vi "NodoPropiedad.vi"() -> ()   [LabVIEW 2015]
uses:
  <vilib>/Utility/miscctls.llb/LVPositionTypeDef.ctl
panel:
  out "Position":T1
  in  "Enum":enum16{"Val1", "Val2", "Val3", "Val4"}(ring)
  in  "Cambiar estado lol":T2(ring)
  out "Estado lol":T2(ring)
  in  "stop":bool
  in  "Ver":bool
  in  "Lol":dbl
  out "xd":bool
  in  "Cual desvisivilizar":bool
  in  "This is a Radio Button":enum32{"Option 1", "Option 2", "Option 3"}(radio)
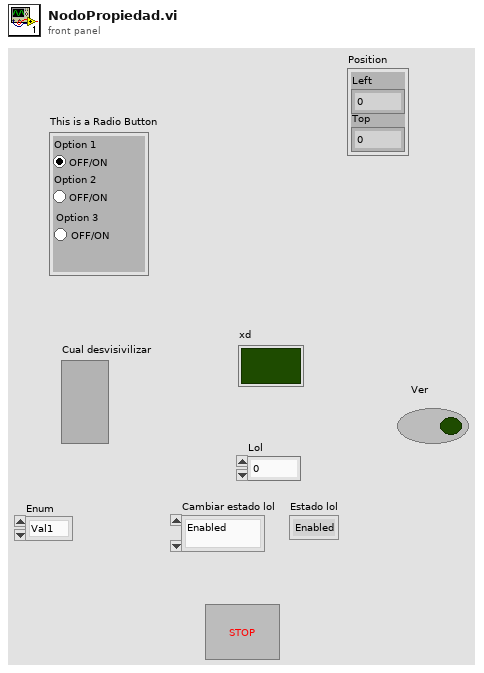
[diagram p1: front panel]
types:
  T1 = typedef "LVPositionTypeDef.ctl" = cluster{"Left":i32, "Top":i32}
  T2 = enum8{"Enabled", "Disabled", "Disabled and Grayed Out"}
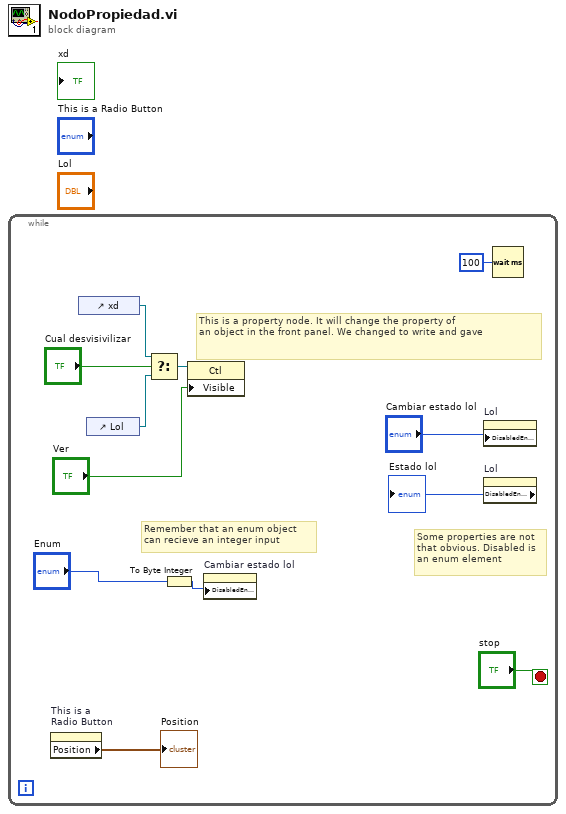
[diagram p0: block diagram]
diagram:
  n1 = while {
    stop <- "stop" stop-if-true
    # "Remember that an enum object \ncan recieve an integer input"
    # "Some properties are not\nthat obvious. Disabled is\nan enum element"
    # "This is a property node. It will change the property of \nan object in the front panel. We changed to write and gave"
    n2 = property on="This is a \nRadio Button" class="RadioBtnsControl (strict)"() -> ("Position"=→"Position":T1)  [unwired: 2 in, 2 out]
    n3 = control-ref of="xd"() -> (w1:refnum<vi>)
    n4 = control-ref of="Lol"() -> (w10:refnum<vi>)
    n5 = Select(t=w1, s="Cual desvisivilizar", f=w10) -> (s? t:f=w8:refnum<vi>)
    n6 = To Byte Integer(number="Enum") -> (8bit integer=w3:i8)
    n7 = property class="Ctl"(reference=w8, "Visible"="Ver") -> ()  [unwired: 1 in, 2 out]
    n8 = property on="Cambiar estado lol" class="Enum (strict)"("DisabledEnum"=w3) -> ()  [unwired: 2 in, 2 out]
    n9 = property on="Lol" class="DigNum (strict)"("DisabledEnum"="Cambiar estado lol") -> ()  [unwired: 2 in, 2 out]
    n10 = property on="Lol" class="DigNum (strict)"() -> ("DisabledEnum"=→"Estado lol":T2)  [unwired: 2 in, 2 out]
    n11 = Wait (ms)(milliseconds to wait=u32 100) -> ()  [unwired: 1 out]
  }
